vi "CRYGet Current Calibration Info.vi"(9 "Is Input?":bool, 11 "Signal Type Name":string) -> (3 "Calibration All Cluster":T1={"Calibration"={"Calibration Step Name"="", "Device"="", "Correction Curve Name"="", "Equalization Curve Name"="", "Sensitivity Curve Name"="", "Corr Folder and File"="", "EQ Folder and File"="", "Sens Folder and File"="", "Corr Step size"=0, "EQ Step size"=0, "Input"=FALSE, "Last Cal Date (sec)"=timestamp(0 s since 1904-01-01), "Cha Name"="", "Corr Curve Found"=FALSE, "EQ Curve Found"=FALSE, "Sens Curve Found"=FALSE, "Signal Type"="", "Calibrated Device"="", "Hz"=0}, "Corr Curve"={"Name"="", "Curve"=[], "X data"=1, "Y data"=1, "Z data"=1, "X axis"=0, "Y axis"=1, "Z axis"=1, "X unit"="", "Y unit"="", "Z unit"="deg.", "X dB ref"=1.0, "Y dB ref"=1.0, "Z dB ref"=1.0, "single val"=FALSE, "protected"=FALSE, "display X"=FALSE, "display Y"=TRUE, "display Z"=TRUE, "Test Info"="", "Step No."=0, "Plot Settings"={"Color"=0, "Interpolation"=0, "Point Style"=0, "Line Style"=0, "Point Color"=0, "Line Width"=0, "Bar Plot Style"=0, "Fill To"=0}, "AutoProtect"=FALSE}, "EQ Curve"={"Name"="", "Curve"=[], "X data"=1, "Y data"=1, "Z data"=1, "X axis"=0, "Y axis"=1, "Z axis"=1, "X unit"="Hz", "Y unit"="", "Z unit"="deg.", "X dB ref"=1.0, "Y dB ref"=1.0, "Z dB ref"=1.0, "single val"=FALSE, "protected"=FALSE, "display X"=TRUE, "display Y"=TRUE, "display Z"=TRUE, "Test Info"="", "Step No."=0, "Plot Settings"={"Color"=0, "Interpolation"=0, "Point Style"=0, "Line Style"=0, "Point Color"=0, "Line Width"=0, "Bar Plot Style"=0, "Fill To"=0}, "AutoProtect"=FALSE}, "Sens Curve"={"Name"="", "Curve"=[], "X data"=1, "Y data"=1, "Z data"=1, "X axis"=0, "Y axis"=1, "Z axis"=1, "X unit"="Hz", "Y unit"="", "Z unit"="deg.", "X dB ref"=1.0, "Y dB ref"=1.0, "Z dB ref"=1.0, "single val"=FALSE, "protected"=FALSE, "display X"=TRUE, "display Y"=TRUE, "display Z"=TRUE, "Test Info"="", "Step No."=0, "Plot Settings"={"Color"=0, "Interpolation"=0, "Point Style"=0, "Line Style"=0, "Point Color"=0, "Line Width"=0, "Bar Plot Style"=0, "Fill To"=0}, "AutoProtect"=FALSE}} {"Sens Curve"."Z data" items=["dB", "Lin"]; "Sens Curve"."X data" items=["dB", "Lin"]; "Sens Curve"."Y data" items=["dB", "Lin"]; "Sens Curve"."Z dB ref" format="%.1f"; "Sens Curve"."Z axis" items=["Log", "Lin"]; "Sens Curve"."X dB ref" format="%.1f"; "Sens Curve"."X axis" items=["Log", "Lin"]; "Sens Curve"."Y axis" items=["Log", "Lin"]; "Sens Curve"."Y dB ref" format="%.1f"; "Sens Curve"."Curve"."z" format="%.2f"; "Sens Curve"."Curve"."y" format="%.2f"; "Sens Curve"."Curve"."x" format="%.2f"; "EQ Curve"."Z data" items=["dB", "Lin"]; "EQ Curve"."X data" items=["dB", "Lin"]; "EQ Curve"."Y data" items=["dB", "Lin"]; "EQ Curve"."Z dB ref" format="%.1f"; "EQ Curve"."Z axis" items=["Log", "Lin"]; "EQ Curve"."X dB ref" format="%.1f"; "EQ Curve"."X axis" items=["Log", "Lin"]; "EQ Curve"."Y axis" items=["Log", "Lin"]; "EQ Curve"."Y dB ref" format="%.1f"; "EQ Curve"."Curve"."z" format="%.2f"; "EQ Curve"."Curve"."y" format="%.2f"; "EQ Curve"."Curve"."x" format="%.2f"; "Corr Curve"."Z data" items=["dB", "Lin"]; "Corr Curve"."X data" items=["dB", "Lin"]; "Corr Curve"."Y data" items=["dB", "Lin"]; "Corr Curve"."Z dB ref" format="%.1f"; "Corr Curve"."Z axis" items=["Log", "Lin"]; "Corr Curve"."X dB ref" format="%.1f"; "Corr Curve"."X axis" items=["Log", "Lin"]; "Corr Curve"."Y axis" items=["Log", "Lin"]; "Corr Curve"."Y dB ref" format="%.1f"; "Corr Curve"."Curve"."z" format="%.2f"; "Corr Curve"."Curve"."y" format="%.2f"; "Corr Curve"."Curve"."x" format="%.2f"; "Calibration"."EQ Step size" items=["R10", "R20", "R40", "R80", "User"]; "Calibration"."Corr Step size" items=["R10", "R20", "R40", "R80", "User"]})   [LabVIEW 2013]
uses:
  Typedef Control/CRYCalibration 2DCluster.ctl
  Typedef Control/CRYCalibration Cluster.ctl
  Typedef Control/CRYData Cluster.ctl
  CRYCal Global.vi
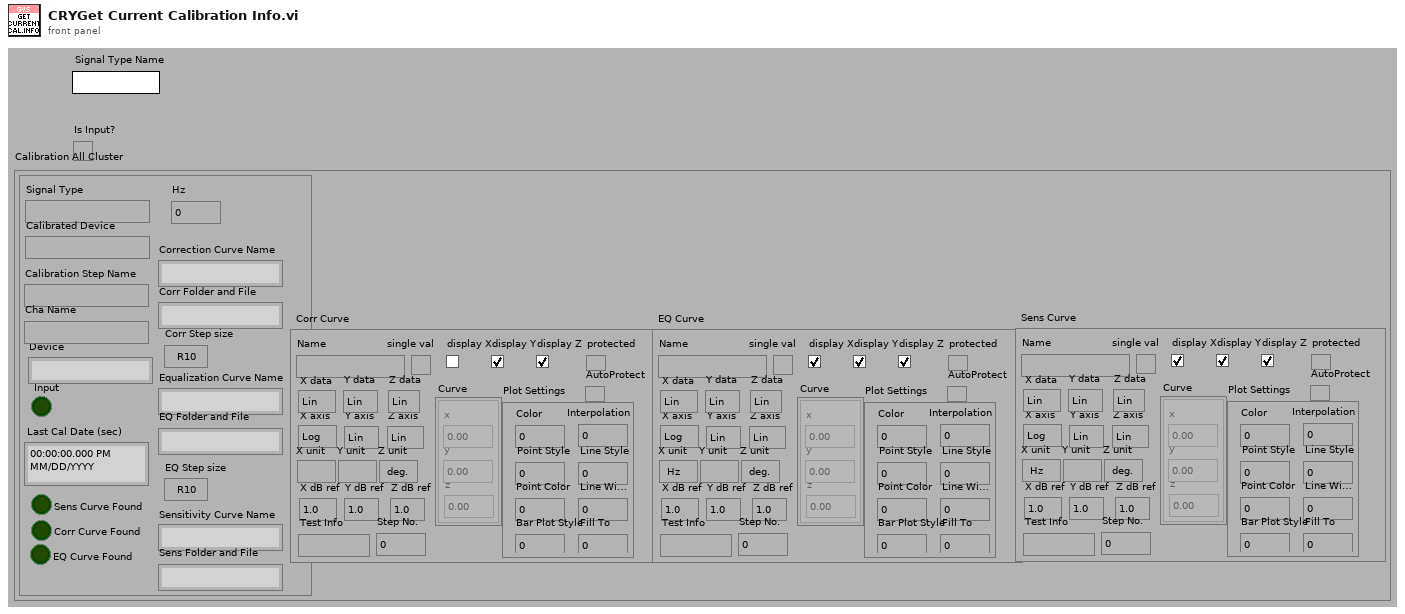
[diagram p1: front panel]
types:
  T1 = typedef "CRYCalibration 2DCluster.ctl" = cluster{"Calibration":T2, "Corr Curve":T3, "EQ Curve":T3, "Sens Curve":T3}
  T2 = typedef "CRYCalibration Cluster.ctl" = cluster{"Calibration Step Name":string, "Device":string, "Correction Curve Name":string, "Equalization Curve Name":string, "Sensitivity Curve Name":string, "Corr Folder and File":string, "EQ Folder and File":string, "Sens Folder and File":string, "Corr Step size":u16, "EQ Step size":u16, "Input":bool, "Last Cal Date (sec)":timestamp, "Cha Name":string, "Corr Curve Found":bool, "EQ Curve Found":bool, "Sens Curve Found":bool, "Signal Type":string, "Calibrated Device":string, "Hz":u32}
  T3 = typedef "CRYData Cluster.ctl" = cluster{"Name":string, "Curve":cluster{"x":dbl, "y":dbl, "z":dbl}[], "X data":u16, "Y data":u16, "Z data":u16, "X axis":u16, "Y axis":u16, "Z axis":u16, "X unit":string, "Y unit":string, "Z unit":string, "X dB ref":dbl, "Y dB ref":dbl, "Z dB ref":dbl, "single val":bool, "protected":bool, "display X":bool, "display Y":bool, "display Z":bool, "Test Info":string, "Step No.":i32, "Plot Settings":cluster{"Color":u32, "Interpolation":u8, "Point Style":u8, "Line Style":u8, "Point Color":u32, "Line Width":u8, "Bar Plot Style":u8, "Fill To":i16}, "AutoProtect":bool}
  T4 = typedef "CRYCalibration All Cluster.ctl" = cluster{"Calibration 2D":T1[], "Help":string, "Tab Value":i32, "Input Signal Type":string, "Output Signal Type":string}
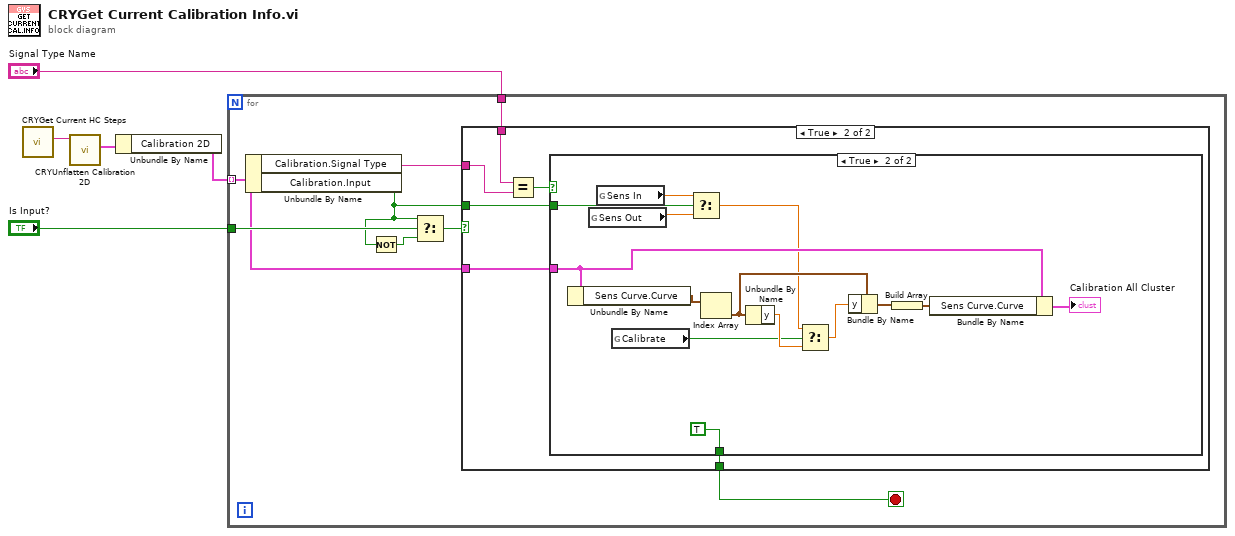
[diagram p0: block diagram]
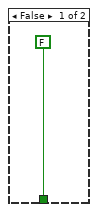
[diagram p2: hidden frame]
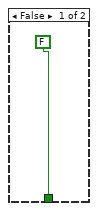
[diagram p3: hidden frame]
diagram:
  n1 = call "CRYGet Current HC Steps.vi"() -> ("Calibration setup flattened Out"=w1:string)  [unwired: 10 in, 1 out]
  n2 = call "CRYUnflatten Calibration 2D.vi"("Flattened Calibration"=w1) -> ("Calibration Step Out"=w3:T4)  [unwired: 10 out]
  n3 = Unbundle By Name(w3) -> ("Calibration 2D"=w2:T1[])
  n4 = for {
    tunnel: w2 -> [w7] mode=indexing
    tunnel: "Is Input?" -> [w13]
    tunnel: "Signal Type Name" -> [w10]
    stop <- w8 stop-if-true
    n5 = Unbundle By Name(w7) -> ("Calibration.Signal Type"=w9:string, "Calibration.Input"=w6:bool)
    n6 = Not(x=w6) -> (.not. x?=w12:bool)
    n7 = Select(t=w6, s=w13, f=w12) -> (s? t:f=w11:bool)
    n8 = case shown="True" w11 {
      tunnel: w10 -> [_ w20]
      tunnel: w9 -> [_ w19]
      tunnel: w7 -> [_ w17]
      tunnel: [FALSE ("stop") w16] -> w8
      tunnel: w6 -> [_ w15]
      frame False {
      }
      frame True {
        n9 = Equal?(x=w20, y=w19) -> (x = y?=w18:bool)
        n10 = case shown="True" w18 {
          tunnel: w17 -> [_ w29]
          tunnel: [FALSE ("stop") TRUE ("stop")] -> w16
          tunnel: w15 -> [_ w26]
          frame False {
          }
          frame True {
            n11 = Unbundle By Name(w29) -> ("Sens Curve.Curve"=w34:cluster{"x":dbl, "y":dbl, "z":dbl}[])
            n12 = global read "CRYCal Global.vi" "Sens Out"() -> (w24:dbl)
            n13 = global read "CRYCal Global.vi" "Sens In"() -> (w25:dbl)
            n14 = global read "CRYCal Global.vi" "Calibrate"() -> (w22:bool)
            n15 = Select(t=w25, s=w26, f=w24) -> (s? t:f=w23:dbl)
            n16 = Index Array(array=w34) -> (element=w32:cluster{"x":dbl, "y":dbl, "z":dbl})  [unwired: 1 in]
            n17 = Unbundle By Name(w32) -> ("y"=w33:dbl)
            n18 = Select(t=w23, s=w22, f=w33) -> (s? t:f=w31:dbl)
            n19 = Bundle By Name(cluster=w32, "y"=w31) -> (w30:cluster{"x":dbl, "y":dbl, "z":dbl})
            n20 = Build Array(w30) -> (w28:cluster{"x":dbl, "y":dbl, "z":dbl}[])
            n21 = Bundle By Name(cluster=w29, "Sens Curve.Curve"=w28) -> (→"Calibration All Cluster":T1)
          }
        }
      }
    }
  }
